vi "hasPacketIdentifier.vi"(11 "PUBLISH in":refnum<class "PUBLISH.lvclass">) -> (2 "As Packet Identifier":bool, 3 "PUBLISH out":refnum<class "PUBLISH.lvclass">)   [LabVIEW 2013, in "PUBLISH.lvclass"]
uses:
  PUBLISH.lvclass
  ControlPacket/ControlPacket.lvclass/ControlPacket.ctl
  ControlPacket/ControlPacket.lvclass
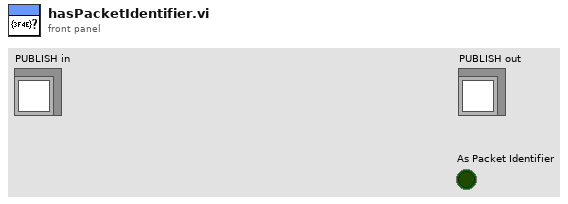
[diagram p1: front panel]
types:
  T1 = typedef "QualityOfService -- enum.ctl" = enum16{"0 (At Most Once)", "1 (At Least Once)", "2 (Exactly Once)"}
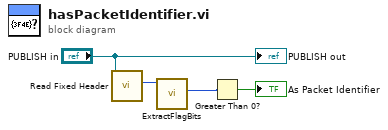
[diagram p0: block diagram]
diagram:
  n1 = call "Read Fixed Header.vi"("ControlPacket in"="PUBLISH in") -> ("Fixed Header"=w3:u8)  [unwired: 9 in, 1 out]
  n2 = call "ExtractFlagBits.vi"("Fixed Header"=w3) -> ("QoS"=w2:T1)  [unwired: 7 in, 3 out]
  n3 = Greater Than 0?(x=w2) -> (x > 0?=→"As Packet Identifier":bool)
  "PUBLISH out" <- "PUBLISH in"
